vi "Path.vi"(8 "error in (no error)":errorcluster, 10 "Path":path, 11 "Generador funciones in":refnum<class "Generador funciones.lvclass">) -> (0 "error out":errorcluster, 3 "Generador funciones out":refnum<class "Generador funciones.lvclass">)   [LabVIEW 2019, in "Generador funciones.lvlib" / "Generador funciones.lvclass"]
uses:
  Generador funciones.lvclass
  Generador funciones.lvclass/Generador funciones.ctl
  Save tdms Messages/Path Msg/Path Msg.lvclass/Path Msg.ctl
  <vilib>/ActorFramework/Message Enqueuer/Message Enqueuer.lvclass/Message Enqueuer.ctl
  Save txt Messages/Path Msg/Path Msg.lvclass/Path Msg.ctl
  <vilib>/ActorFramework/Message Enqueuer/Enqueue.vi
  Save tdms Messages/Path Msg/Path Msg.lvclass
  C:/Program Files/National Instruments/LabVIEW 2019/vi.lib/ActorFramework/Message/Message.lvclass
  Save txt Messages/Path Msg/Path Msg.lvclass
  <vilib>/ActorFramework/Message Priority Queue/Priority Enqueue.vi
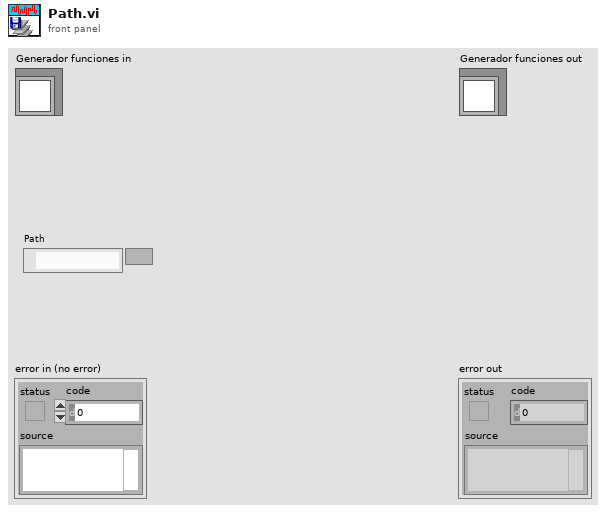
[diagram p1: front panel]
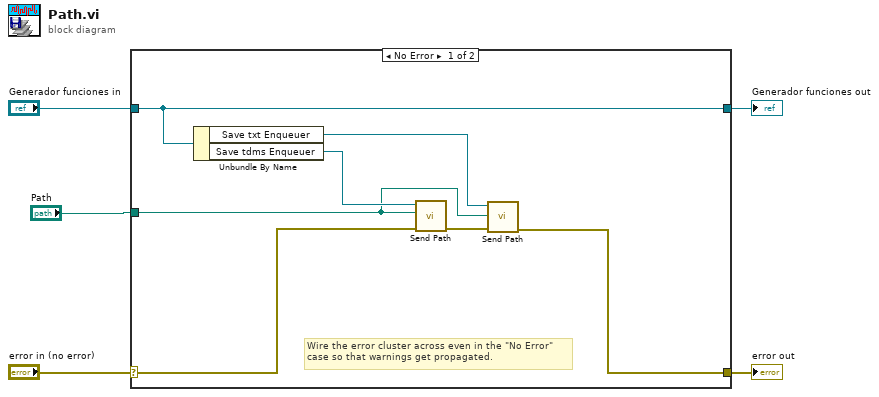
[diagram p0: block diagram]
diagram:
  n1 = case shown="No Error" "error in (no error)" {
    selector: "error in (no error)" -> [w7 w14]
    tunnel: [w6 w14] -> w4
    tunnel: [w12 w13] -> w2
    tunnel: "Generador funciones in" -> [w12 w13]
    tunnel: "Path" -> [w9 _]
    frame No Error {
      # "Wire the error cluster across even in the \"No Error\"\ncase so that warnings get propagated."
      n2 = Unbundle By Name(w12) -> ("Save txt Enqueuer"=w10:refnum<class "Message Enqueuer.lvclass">, "Save tdms Enqueuer"=w11:refnum<class "Message Enqueuer.lvclass">)
      n3 = call "Send Path.vi"("error in (no error)"=w7, "Path"=w9, "Message Enqueuer"=w11) -> ("error out"=w8:errorcluster)  [unwired: 7 in, 1 out]
      n4 = call "Send Path.vi"("error in (no error)"=w8, "Path"=w9, "Message Enqueuer"=w10) -> ("error out"=w6:errorcluster)  [unwired: 7 in, 1 out]
    }
    frame Error {
    }
  }
  "error out" <- w4
  "Generador funciones out" <- w2
